vi "DFConfig Remove Datafinder Run Key.vi"(8 "error in (no error)":errorcluster) -> (0 "error out":errorcluster)   [LabVIEW 2011]
uses:
  <vilib>/registry/registry.llb/Registry RtKey.ctl
panel:
  out "subkeys":string[](array[string])
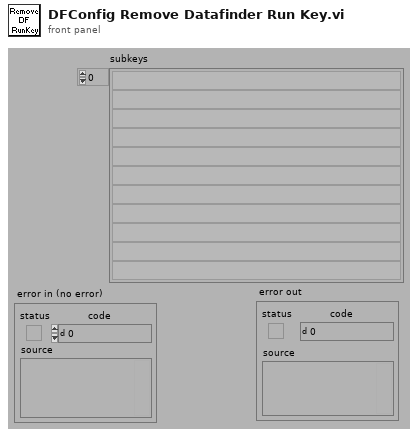
[diagram p1: front panel]
types:
  T1 = typedef "Registry RtKey.ctl" = enum32{"HKEY_CLASSES_ROOT", "HKEY_CURRENT_USER", "HKEY_LOCAL_MACHINE", "HKEY_USERS", "HKEY_PERFORMANCE_DATA", "HKEY_CURRENT_CONFIG", "HKEY_DYN_DATA"}
  T2 = typedef "Registry refnum.ctl" = refnum<k1>
  T3 = cluster{"numValues":i32, "maxValueNameLen":i32, "maxValueDataLen":i32}
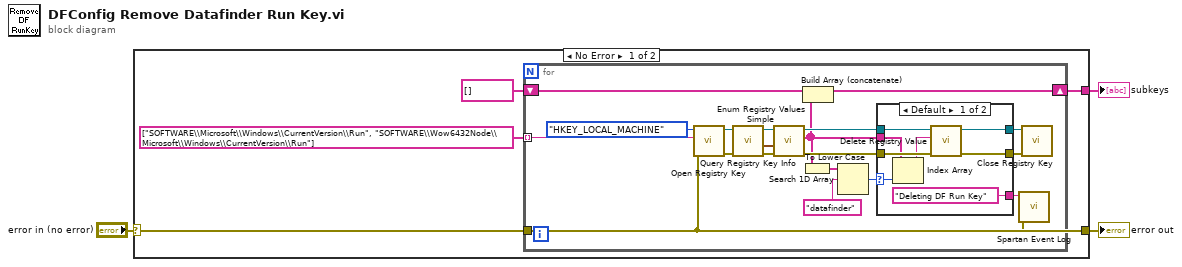
[diagram p0: block diagram]
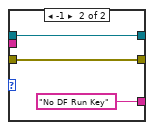
[diagram p2: hidden frame]
diagram:
  n1 = case shown="No Error" "error in (no error)" {
    selector: "error in (no error)" -> [w7 w38]
    tunnel: [w4 _] -> w3
    tunnel: [w7 w38] -> w1
    frame No Error {
      n2 = for {
        tunnel: w7 -> [w13]
        tunnel: string[] ["SOFTWARE\\Microsoft\\Windows\\CurrentVersion\\Run", "SOFTWARE\\Wow6432Node\\Microsoft\\Windows\\CurrentVersion\\Run"] -> [w11] mode=indexing
        shift-right: [w9] -> w4
        shift-left: string[] [] -> [w10]
        n3 = call <vilib>:"Open Registry Key.vi"("error in (no error)"=w13, "subkey"=w11, "root key (HKEY_LOCAL_MACHINE)"=Registry_RtKey."HKEY_LOCAL_MACHINE") -> ("error out"=w23:errorcluster, "refnum out"=w25:T2)  [unwired: 7 out]
        n4 = call <vilib>:"Query Registry Key Info.vi"("error in (no error)"=w23, "refnum"=w25) -> ("error out"=w22:errorcluster, "value info"=w21:T3, "refnum out"=w24:T2)  [unwired: 7 out]
        n5 = call <vilib>:"Enum Registry Values Simple.vi"("error in (no error)"=w22, "value info"=w21, "refnum"=w24) -> ("error out"=w17:errorcluster, "values"=w8:string[], "refnum out"=w18:T2)  [unwired: 1 in, 5 out]
        n6 = To Lower Case(string=w8) -> (all lower case string=w20:string[])
        n7 = Build Array (concatenate)(w10, w8) -> (w9:string[])
        n8 = Search 1D Array(1D array=w20, element="datafinder") -> (index of element=w12:i32)  [unwired: 1 out]
        n9 = case shown="Default" w12 {
          selector: w12 -> [w27 _]
          tunnel: w18 -> [w34 w36]
          tunnel: w17 -> [w32 w37]
          tunnel: [w31 w37] -> w16
          tunnel: [w33 w36] -> w15
          tunnel: w8 -> [w30 _]
          tunnel: ["Deleting DF Run Key" ("module (\"\")") "No DF Run Key" ("module (\"\")")] -> w14
          frame Default {
            n10 = Index Array(array=w30, index=w27) -> (element=w29:string)
            n11 = call <vilib>:"Delete Registry Value.vi"("error in (no error)"=w32, "value"=w29, "refnum"=w34) -> ("error out"=w31:errorcluster, "refnum out"=w33:T2)  [unwired: 7 out]
          }
          frame -1 {
          }
        }
        n12 = call "Spartan Event Log.vi"("error in (no error)"=w13, "message (\"\")"=w14) -> ()  [unwired: 3 in, 4 out]
        n13 = call <vilib>:"Close Registry Key.vi"("error in (no error)"=w16, "refnum"=w15) -> ()  [unwired: 6 out]
      }
    }
    frame Error {
    }
  }
  "error out" <- w1
  "subkeys" <- w3
